vi "stage step to next field.vi"(1 "# Fields across x":i8(slide)=3 min=1 max=10 step=1 scale=0.0..10.0, 2 "Go":bool, 3 "Initialize":bool=TRUE, 4 "# Fields across y":i8(slide)=3 min=1 max=10 step=1 scale=0.0..10.0, 5 "error in (no error)":errorcluster) -> (8 "error out":errorcluster)   [LabVIEW 2015]
doc: "This VI is used to scan the stage through a rectangular array of fields. The x and y dimensions are always the maximum scan dimensions of the stage, which are set in Stage Globals.vi\n\nWhen called in initialize mode, allows the user to interactively select the x and y dimensions of the rectangular array. When selection is complete, the user should press go.\n\nWhen called with initialize = false (ordinarily, non-interactively), steps the stage to the next position in the array. The array is scanned in a raster fashion, with x movements more frequent and y more rare."
uses:
  Move stage command.ctl
  new-h-nu-ixon/stage globals.vi
  stage step to next field globals.vi
panel:
  in  "Stage settle time (ms)":u32=2000
  out "Stage Positions":cluster{dbl, dbl}[](graph)
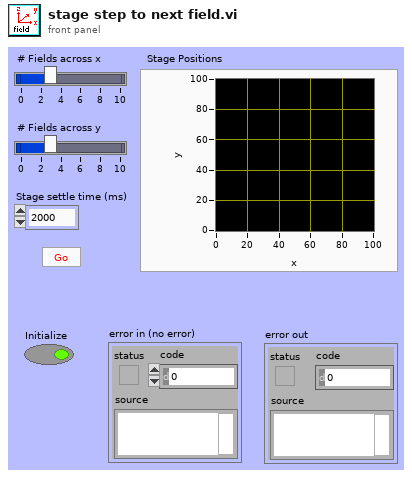
[diagram p1: front panel]
types:
  T1 = enum32{"Invalid", "Standard", "Closed", "Hidden", "Minimized", "Maximized"}
  T2 = typedef "Move stage command.ctl" = cluster{"dx (um) (0 -> ignore)":ext, "dy (um) (0 -> ignore)":ext, "dz (um) (0 -> ignore)":ext, "Re-center x,y":bool, "Re-center z":bool, "x (um) (-1 -> ignore)":dbl, "y (um) (-1 -> ignore)":dbl, "z (um) (-1 -> ignore)":dbl}
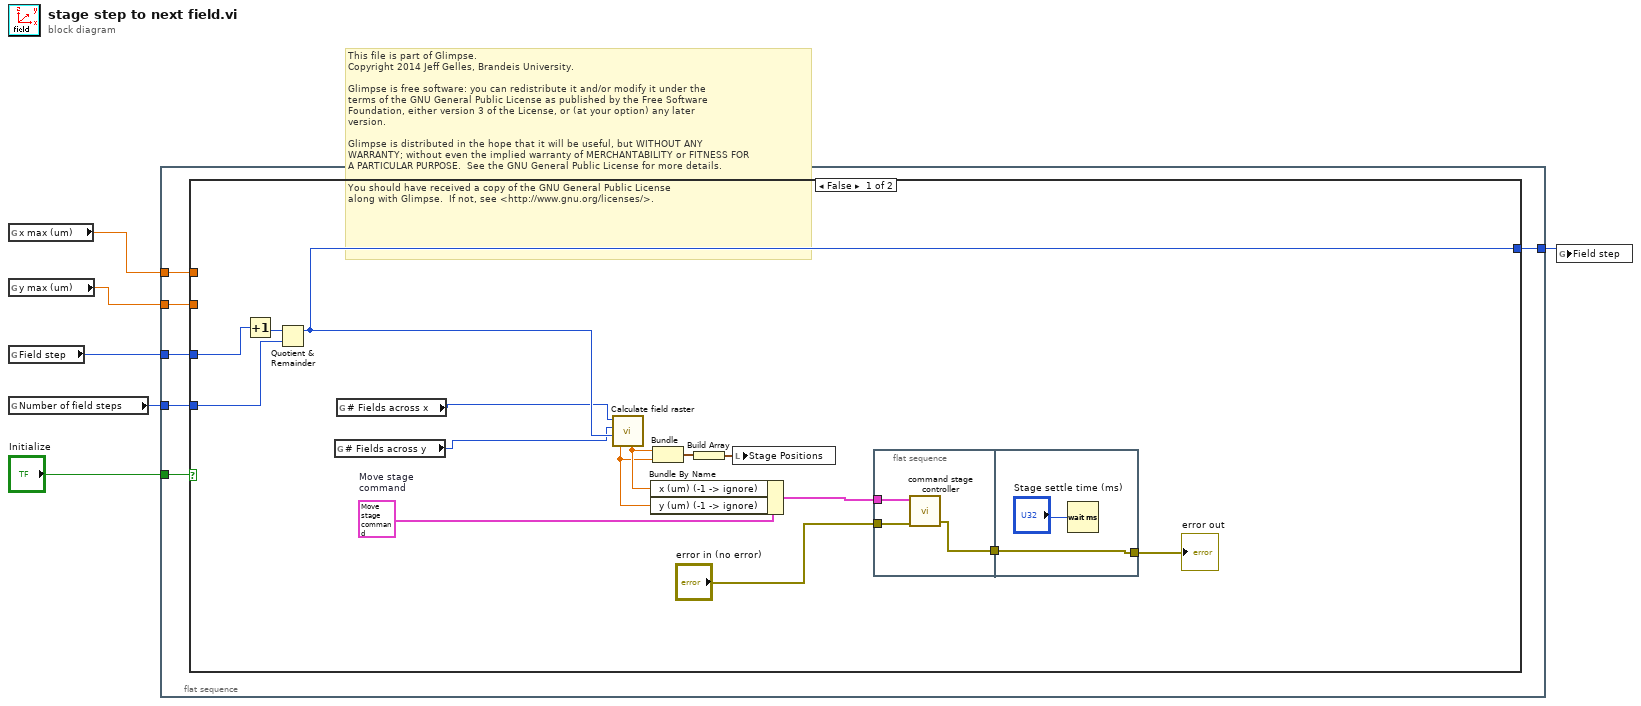
[diagram p0: block diagram]
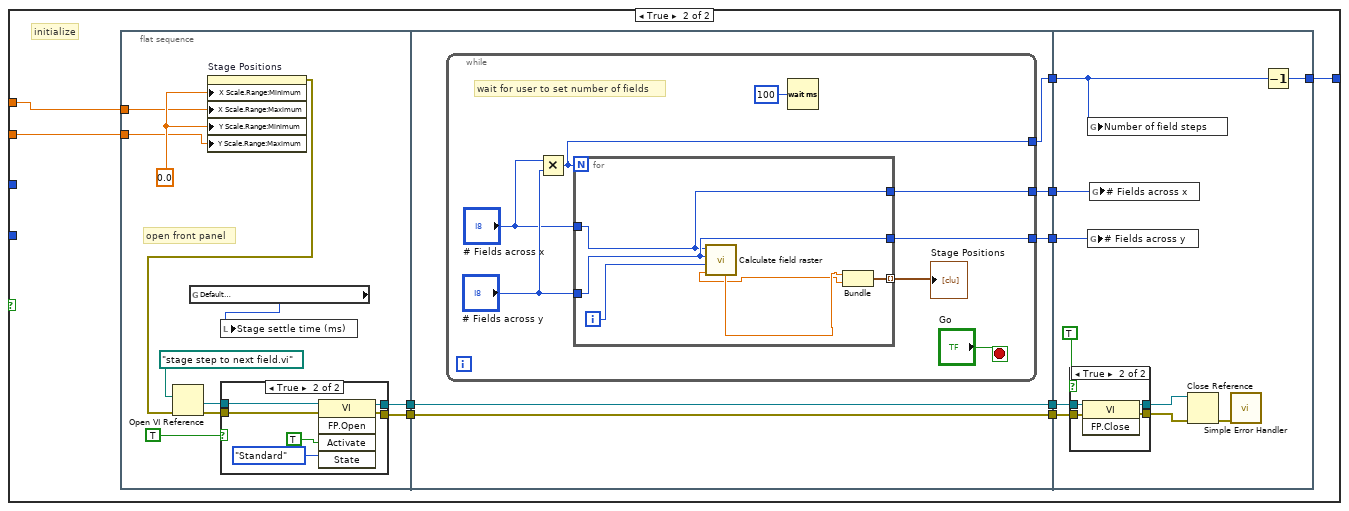
[diagram p2: hidden frame]
diagram:
  # "This file is part of Glimpse. \nCopyright 2014 Jeff Gelles, Brandeis University.    \n\nGlimpse is free software: you can redistribute it and/or modify it under the \nterms of the GNU General Public License as published by the Free Software \nFoundation, either version 3 of the License, or (at your option) any later \nversion.\n\nGlimpse is distributed in the hope that it will be useful, but WITHOUT ANY \nWARRANTY; without even the implied warranty of MERCHANTABILITY or FITNESS FOR \nA PARTICULAR PURPOSE.  See the GNU General Public License for more details.\n\nYou should have received a copy of the GNU General Public License\nalong with Glimpse.  If not, see <http://www.gnu.org/licenses/>."
  n1 = global read "stage globals.vi" "x max (um)"() -> (w4:ext)
  n2 = global read "stage globals.vi" "y max (um)"() -> (w1:ext)
  n3 = global read "stage globals.vi" "Field step"() -> (w5:i16)
  n4 = global read "stage globals.vi" "Number of field steps"() -> (w3:i16)
  n5 = flat-sequence {
    tunnel: [w8] -> w2
    tunnel: "Initialize" -> [w12]
    tunnel: w5 -> [w11]
    tunnel: w4 -> [w10]
    tunnel: w3 -> [w9]
    tunnel: w1 -> [w7]
    frame #0 {
      n6 = case shown="False" w12 {
        tunnel: [w25 w41] -> w8
        tunnel: w11 -> [w23 _]
        tunnel: w10 -> [_ w36]
        tunnel: w9 -> [w22 _]
        tunnel: w7 -> [_ w35]
        frame False {
          w20 = T2 {"dx (um) (0 -> ignore)"=0.0, "dy (um) (0 -> ignore)"=0.0, "dz (um) (0 -> ignore)"=0.0, "Re-center x,y"=FALSE, "Re-center z"=FALSE, "x (um) (-1 -> ignore)"=-1.0, "y (um) (-1 -> ignore)"=-1.0, "z (um) (-1 -> ignore)"=-1.0}  # Move stage command
          n7 = Increment(x=w23) -> (x+1=w24:i16)
          n8 = Quotient & Remainder(x=w24, y=w22) -> (x-y*floor(x/y)=w25:i16)  [unwired: 1 out]
          n9 = global read "stage step to next field globals.vi" "# Fields across y"() -> (w14:i8)
          n10 = global read "stage step to next field globals.vi" "# Fields across x"() -> (w13:i8)
          n11 = call "Calculate field raster.vi"("# Fields across x"=w13, "# Fields across y"=w14, "Index (0 to n-1)"=w25) -> ("y"=w18:dbl, "x"=w19:dbl)  [unwired: 1 in, 4 out]
          n12 = Bundle By Name(cluster=w20, "x (um) (-1 -> ignore)"=w19, "y (um) (-1 -> ignore)"=w18) -> (w21:T2)
          n13 = Bundle("x"=w19, "y"=w18) -> (w27:cluster{"x":dbl, "y":dbl})  [unwired: 1 out]
          n14 = Build Array(w27) -> (w26:cluster{"x":dbl, "y":dbl}[])
          n15 = local write "Stage Positions"(w26) -> ()
          n16 = flat-sequence {
            tunnel: w21 -> [w30]
            tunnel: "error in (no error)" -> [w29]
            tunnel: [w28] -> w15
            tunnel: [w31] -> w16
            tunnel: w15 -> [w31]
            frame #0 {
              n17 = call "command stage controller.vi"("command"=w30, "error in (no error)"=w29) -> ("error out"=w28:errorcluster)  [unwired: 6 out]
            }
            frame #1 {
              n18 = Wait (ms)(milliseconds to wait="Stage settle time (ms)") -> ()  [unwired: 1 out]
            }
          }
          "error out" <- w16
        }
        frame True {
          # "initialize"
          n19 = flat-sequence {
            tunnel: w35 -> [w47]
            tunnel: [w50] -> w40
            tunnel: [w49] -> w37
            tunnel: w36 -> [w43]
            tunnel: [w66] -> w42
            tunnel: w40 -> [w65]
            tunnel: [w65] -> w39
            tunnel: [w64] -> w38
            tunnel: w37 -> [w64]
            tunnel: [w63] -> w34
            tunnel: [w62] -> w33
            tunnel: w42 -> [w89]
            tunnel: [w90] -> w41
            tunnel: w39 -> [w87]
            tunnel: w38 -> [w86]
            tunnel: w34 -> [w82]
            tunnel: w33 -> [w81]
            frame #0 {
              w48 = 0.0 ("X Scale.Range:Minimum")
              # "open front panel"
              n20 = global read "stage globals.vi" "Default\nstage settle time (ms)"() -> (w44:u32)
              n21 = property on="Stage Positions" class="XYGraph (strict)"("X Scale.Range:Minimum"=w48, "X Scale.Range:Maximum"=w43, "Y Scale.Range:Minimum"=w48, "Y Scale.Range:Maximum"=w47) -> (error out=w46:errorcluster)  [unwired: 2 in, 1 out]
              n22 = Open VI Reference(vi path=path "stage step to next field.vi", error in (no error)=w46) -> (vi reference=w51:refnum<vi>, error out=w52:errorcluster)  [unwired: 4 out]
              n23 = local write "Stage settle time (ms)"(w44) -> ()
              n24 = case shown="True" TRUE ("Case Constant\n(See Context Help)") {
                tunnel: w52 -> [w55 w61]
                tunnel: w51 -> [w54 w60]
                tunnel: [w54 w57] -> w50
                tunnel: [w55 w56] -> w49
                frame False {
                }
                frame True {
                  n25 = invoke class="VI" method="FP.Open"(reference=w60, error in=w61, "Activate"=TRUE, "State"=T1."Standard") -> (reference out=w57:refnum<vi>, error out=w56:errorcluster)  [unwired: 1 in, 3 out]
                }
              }
            }
            frame #1 {
              n26 = while {
                tunnel: [w69] -> w66
                tunnel: [w68] -> w63
                tunnel: [w67] -> w62
                stop <- "Go" stop-if-true
                # "wait for user to set number of fields"
                n27 = Multiply(x="# Fields across x", y="# Fields across y") -> (x*y=w69:i8)
                n28 = for {
                  N: w69 -> [_]
                  tunnel: "# Fields across y" -> [w76]
                  tunnel: "# Fields across x" -> [w75]
                  tunnel: [w77] -> w71 mode=indexing
                  tunnel: [w76] -> w68
                  tunnel: [w75] -> w67
                  i -> [w80]
                  n29 = call "Calculate field raster.vi"("# Fields across x"=w75, "# Fields across y"=w76, "Index (0 to n-1)"=w80) -> ("y"=w78:dbl, "x"=w79:dbl)  [unwired: 1 in, 4 out]
                  n30 = Bundle("x"=w79, "y"=w78) -> (w77:cluster{"x":dbl, "y":dbl})  [unwired: 1 out]
                }
                "Stage Positions" <- w71
                n31 = Wait (ms)(milliseconds to wait=u32 100) -> ()  [unwired: 1 out]
              }
            }
            frame #2 {
              n32 = case shown="True" TRUE ("Case Constant\n(See Context Help) 2") {
                tunnel: w87 -> [w92 w96]
                tunnel: w86 -> [w91 w95]
                tunnel: [w91 w94] -> w85
                tunnel: [w92 w93] -> w84
                frame False {
                }
                frame True {
                  n33 = invoke class="VI" method="FP.Close"(reference=w96, error in=w95) -> (reference out=w93:refnum<vi>, error out=w94:errorcluster)  [unwired: 1 in, 1 out]
                }
              }
              n34 = global write "stage globals.vi" "Number of field steps"(w89) -> ()
              n35 = global write "stage step to next field globals.vi" "# Fields across y"(w82) -> ()
              n36 = global write "stage step to next field globals.vi" "# Fields across x"(w81) -> ()
              n37 = Close Reference(reference=w84, error in (no error)=w85) -> (error out=w88:errorcluster)
              n38 = call <vilib>:"Simple Error Handler.vi"("error in (no error)"=w88) -> ()  [unwired: 1 in, 8 out]
              n39 = Decrement(x=w89) -> (x-1=w90:i8)
            }
          }
        }
      }
    }
  }
  n40 = global write "stage globals.vi" "Field step"(w2) -> ()
